vi "rs3 stop 3.vi"(8 "error in (no error)":errorcluster, 11 "sensor":u64) -> (0 "error out":errorcluster, 2 "sensor out":u64, 3 "error":u64)   [LabVIEW 2019, in "libRealSense3.lvlib"]
doc: "Stops streaming on the specified sensor."
uses:
  libRealSense3.lvlib
  realsense2.dll
panel:
  # "RS3 Stop"
  # "(C) Intel Corp. 2017,  AGJ"
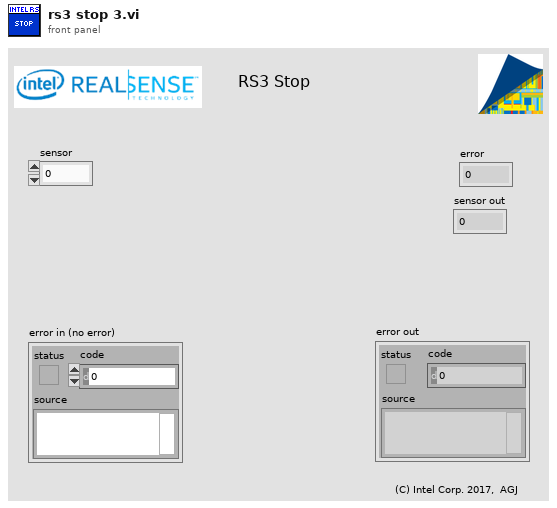
[diagram p1: front panel]
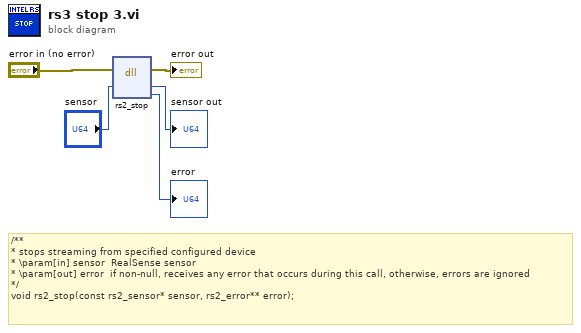
[diagram p0: block diagram]
diagram:
  # "/**\n* stops streaming from specified configured device\n* \\param[in] sensor  RealSense sensor\n* \\param[out] error  if non-null, receives any error that occurs during this call, otherwise, errors are ignored\n*/\nvoid rs2_stop(const rs2_sensor* sensor, rs2_error** error);"
  n1 = dll-call lib="C:/Users/morte/Documents/gitmoro/treadmill/RealSense for Labview ver. 2.33/realsense2.dll" fn="rs2_stop"(error in="error in (no error)", "device"="sensor") -> (error out=→"error out":errorcluster, "device"=→"sensor out":u64, "error"=→"error":u64)  [unwired: 4 in, 1 out]
